vi "Sync Major Frame Messages.vi"(7 "Minor Frame":refnum<class "Minor Frame.lvclass">, 8 "error in (no error)":errorcluster, 11 "Major Frame in":refnum<class "Major Frame.lvclass">) -> (0 "error out":errorcluster, 3 "Major Frame out":refnum<class "Major Frame.lvclass">)   [LabVIEW 2020, in "BCI-1553 API.lvlib" / "Major Frame.lvclass"]
doc: "Called after a minor frame has been configured.\n\nUpdates the Major Frame message table. This makes sure that we have no duplicated message definitions after configuring a minor frame."
uses:
  Major Frame.lvclass
  Minor Frame/Minor Frame.lvclass
  Major Frame.lvclass/Major Frame.ctl
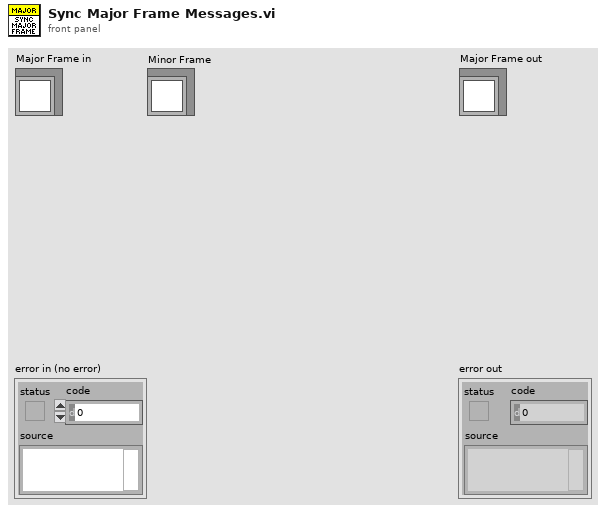
[diagram p1: front panel]
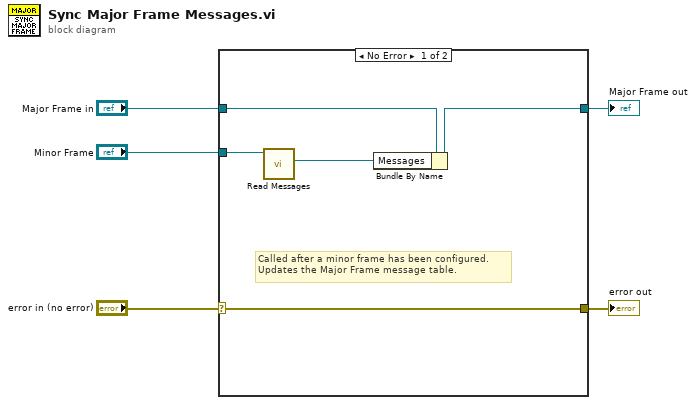
[diagram p0: block diagram]
diagram:
  n1 = case shown="No Error" "error in (no error)" {
    selector: "error in (no error)" -> [w10 w12]
    tunnel: [w10 w12] -> w4
    tunnel: [w7 w11] -> w2
    tunnel: "Major Frame in" -> [w8 w11]
    tunnel: "Minor Frame" -> [w9 _]
    frame No Error {
      # "Called after a minor frame has been configured.\nUpdates the Major Frame message table."
      n2 = call-dynamic "Read Messages.vi"("Minor Frame in"=w9) -> ("Messages"=w6:refnum<class "Registry.lvclass">)  [unwired: 8 in, 2 out]
      n3 = Bundle By Name(cluster=w8, "Messages"=w6) -> (w7:refnum<class "Major Frame.lvclass">)
    }
    frame Error {
    }
  }
  "error out" <- w4
  "Major Frame out" <- w2
